vi "String Move Last TopLevelDiagram declarations to begin.vi"(1 "C code in":string) -> (0 "C code modified":string)   [LabVIEW 2014]
uses:
  <vilib>/regexp/Match Regular Expression.xnode
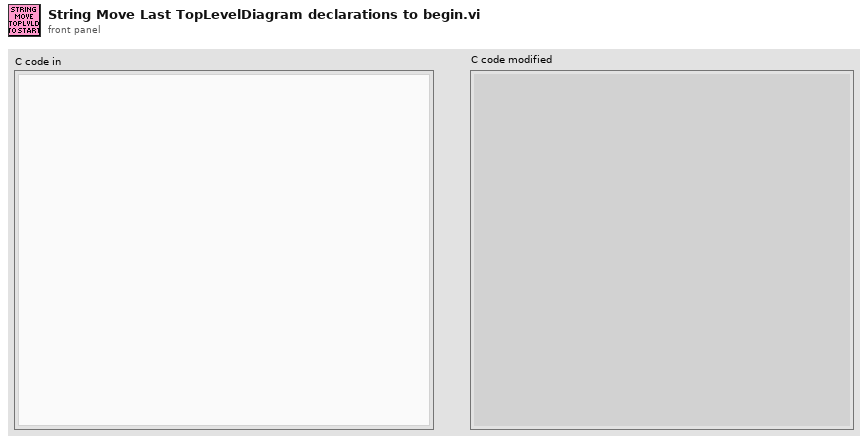
[diagram p1: front panel]
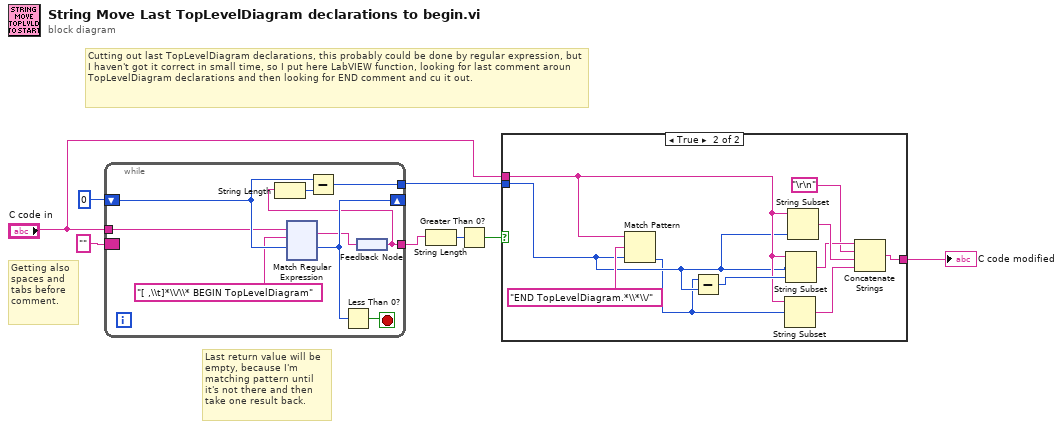
[diagram p0: block diagram]
diagram:
  # "Getting also spaces and tabs before comment."
  # "Last return value will be empty, because I'm matching pattern until it's not there and then take one result back."
  # "Cutting out last TopLevelDiagram declarations, this probably could be done by regular expression, but I haven't got it correct in small time, so I put here LabVIEW function, looking for last comment aroun TopLevelDiagram declarations and then looking for END comment and cu it out."
  n1 = while {
    tunnel: "C code in" -> [w11]
    shift-right: [w13] -> _
    shift-left: 0 ("offset past match") -> [w16]
    tunnel: [w9] -> w5
    tunnel: [w15] -> w4
    border: "" ("C code in") -> [_]
    stop <- w17 stop-if-true
    n2 = xnode "Match Regular Expression"("input string"=w11, "regular expression"="[ ,\\t]*\\/\\* BEGIN TopLevelDiagram", "offset (0)"=w16) -> ("whole match"=w10:string, "offset past match"=w13:i32)  [unwired: 3 in, 3 out]
    n3 = Less Than 0?(x=w13) -> (x < 0?=w17:bool)
    n4 = feedback-in #1(w10) -> ()
    n5 = feedback #1() -> (w9:string)
    n6 = String Length(string=w9) -> (length=w14:i32)
    n7 = Subtract(x=w16, y=w14) -> (x-y=w15:i32)
  }
  n8 = String Length(string=w5) -> (length=w7:i32)
  n9 = Greater Than 0?(x=w7) -> (x > 0?=w6:bool)
  n10 = case shown="True" w6 {
    tunnel: w4 -> [_ w136]
    tunnel: "C code in" -> [w132 w137]
    tunnel: [w132 w138] -> w1
    frame False {
    }
    frame True {
      n11 = Match Pattern(string=w137, regular expression="END TopLevelDiagram.*\\*\\/", offset (0)=w136) -> (offset past match=w135:i32)  [unwired: 3 out]
      n12 = Subtract(x=w135, y=w136) -> (x-y=w141:i32)
      n13 = String Subset(string=w137, offset (0)=w135) -> (substring=w139:string)  [unwired: 1 in]
      n14 = String Subset(string=w137, offset (0)=w136, length (rest)=w141) -> (substring=w134:string)
      n15 = String Subset(string=w137, length (rest)=w136) -> (substring=w140:string)  [unwired: 1 in]
      n16 = Concatenate Strings(w134, "\r\n", w140, w139) -> (w138:string)
    }
  }
  "C code modified" <- w1
